vi "Get Subaddress Endpoint.vi"(8 "error in":errorcluster, 11 "subaddress":T1 format="%.0x") -> (0 "error out":errorcluster, 2 "remote terminal endpoint":T2, 3 "subaddress out":T1 format="%.0x")   [LabVIEW 2020, in "AIM MIL-STD-1553 Scripting.lvlib"]
doc: "Returns the <b>endpoint</b> (terminal address and subaddress) for the parent remote terminal of the <b>subaddress</b>."
uses:
  AIM MIL-STD-1553 Scripting.lvlib
  <vilib>/NI VeriStand/Custom Device API/Custom Device Item Ref.ctl
  Shared/Terminal Endpoint.ctl
  Shared/Address.ctl
  <vilib>/NI VeriStand/Custom Device API/Custom Device API.lvlib
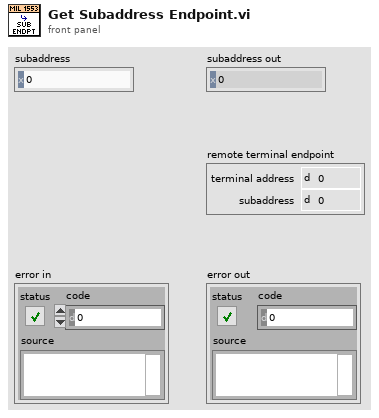
[diagram p1: front panel]
types:
  T1 = typedef "Custom Device API.lvlib/Custom Device Item Ref.ctl" = u64
  T2 = typedef "Terminal Endpoint.ctl" = cluster{"terminal address":T3, "subaddress":T3}
  T3 = typedef "Address.ctl" = u16
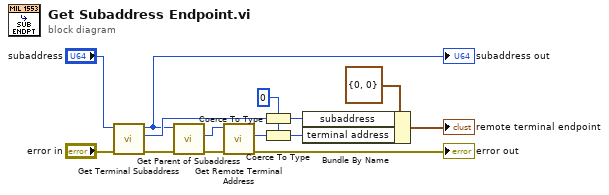
[diagram p0: block diagram]
diagram:
  w6 = T3 0 ("subaddress")
  n1 = call "Get Terminal Subaddress.vi"("error in"="error in", "subaddress section"="subaddress") -> ("error out"=w4:errorcluster, "subaddress value"=w10:T3, "subaddress section out"=w1:T1)  [unwired: 6 in, 1 out]
  "subaddress out" <- w1
  n2 = call "Get Parent of Subaddress.vi"("error in"=w4, "subaddress"=w1) -> ("error out"=w3:errorcluster, "parent of subaddress"=w2:T1)  [unwired: 7 in, 1 out]
  n3 = call "Get Remote Terminal Address.vi"("error in"=w3, "remote terminal"=w2) -> ("error out"=→"error out":errorcluster, "terminal address"=w8:T3)  [unwired: 6 in, 2 out]
  n4 = Coerce To Type(0:w10, 1:w6) -> (2:w9:T3)
  n5 = Coerce To Type(0:w8, 1:w6) -> (2:w7:T3)
  n6 = Bundle By Name(cluster=T2 {"terminal address"=0, "subaddress"=0} ("endpoint Rx"), "subaddress"=w9, "terminal address"=w7) -> (→"remote terminal endpoint":T2)
